vi "Read Size.vi"(8 "Error In":errorcluster, 11 "SFTP File In":refnum<class "SFTP File.lvclass">) -> (0 "Error Out":errorcluster, 2 "File Size":u64, 3 "SFTP File Out":refnum<class "SFTP File.lvclass">)   [LabVIEW 2018, in "Toolkit.lvlib" / "SFTP File.lvclass"]
uses:
  SFTP File.lvclass
  SFTP Attributes/SFTP Attributes.lvclass/SFTP Attributes.ctl
  SSH/SSH.lvclass/SSH.ctl
  SSH/Utility/Read Shared Library.vi
  SFTP Attributes/Support/Create from SFTP File.vi
  Support/Check Status.vi
  SFTP Attributes/Support/Destroy to SFTP File.vi
  SFTP Attributes/SFTP Attributes.lvclass
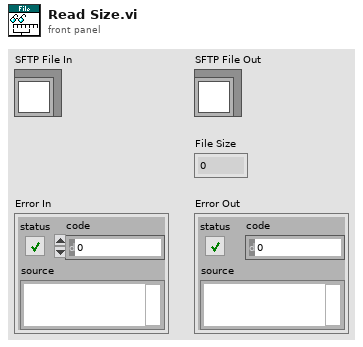
[diagram p1: front panel]
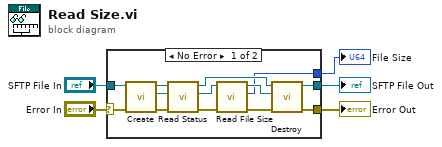
[diagram p0: block diagram]
diagram:
  n1 = case shown="No Error" "Error In" {
    selector: "Error In" -> [w10 w19]
    tunnel: "SFTP File In" -> [w9 w20]
    tunnel: [w8 w20] -> w2
    tunnel: [w7 w19] -> w3
    tunnel: [w6 _] -> w1
    frame No Error {
      n2 = call-poly "Create.vi"("Error In"=w10, "SFTP File In"=w9) -> ("Error Out"=w11:errorcluster, "SFTP Attributes"=w17:refnum<class "SFTP Attributes.lvclass">, "SFTP File Out"=w18:refnum<class "SFTP File.lvclass">)  [unwired: 7 in]
      n3 = call "Read Status.vi"("Error In"=w11, "Attributes In"=w17, "SFTP File In"=w18) -> ("Error Out"=w15:errorcluster, "Attributes Out"=w16:refnum<class "SFTP Attributes.lvclass">, "SFTP File Out"=w14:refnum<class "SFTP File.lvclass">)  [unwired: 6 in]
      n4 = call "Read File Size.vi"("Error In"=w15, "SFTP Attributes In"=w16) -> ("Error Out"=w12:errorcluster, "File Size"=w6:u64, "SFTP Attribute Out"=w13:refnum<class "SFTP Attributes.lvclass">)  [unwired: 7 in]
      n5 = call-poly "Destroy.vi"("Error In"=w12, "SFTP Attributes"=w13, "SFTP File In"=w14) -> ("Error Out"=w7:errorcluster, "SFTP File Out"=w8:refnum<class "SFTP File.lvclass">)  [unwired: 7 in]
    }
    frame Error {
    }
  }
  "Error Out" <- w3
  "SFTP File Out" <- w2
  "File Size" <- w1
